vi "WriteLogFile.vi"(4 "Run uninterrupted?":bool, 6 "Automatic warning":string caption="Automatic warning (e.g. large Temperature/RH fluctuations)", 7 "Data File":string, 8 "Error In":errorcluster, 9 "DUT passed?":bool, 10 "Value TechSpec criteria":dbl, 11 "Files saved?":bool) -> (0 "Error Out":errorcluster)   [LabVIEW 2018]
uses:
  globals/QC_RunInformation.vi
panel:
  out "Cause for quitting measurement":string
  in  "OK Button":bool
  in  "Add comment":bool
  out "Type of measurement":string
  out "Logfile entry":string
  # "Write Logfile"
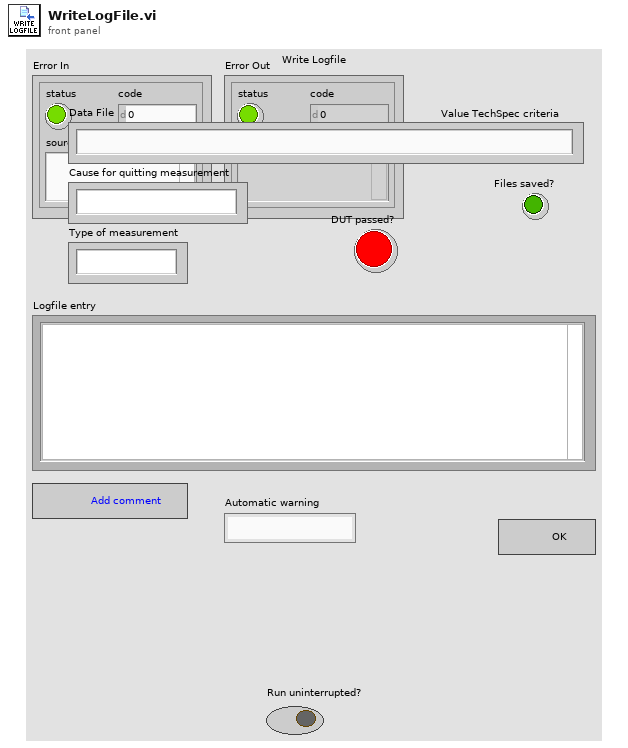
[diagram p1: front panel]
types:
  T1 = enum16{"open", "replace", "create", "open or create", "replace or create", "replace or create with confirmation"}
  T2 = cluster{"Sensor Serial No.:":string, "Wafer:":string, "Batch:":string, "Manufacturer:":string, "Device Category:":string, "Database Serial No.:":string, "Date Initiated:":string, "Time Initiated:":string, "Test":string, "Probeplan used:":string, "End of Run Status":dbl, "End of Run comment:":string, "User:":string, "Vbias SMU":string, "LCR":string, "Test SMU":string, "Test DMM":string, "Comments":string, "Measurement results":cluster{"IV":string, "CV":string, "Cis":string, "Ris":string, "Stability":string, "PTP":string, "Striptest":string}}
  T3 = cluster{"Institute":string, "Manufacturers":string[], "Devices":string[], "Serialnumbers Lookup DB":string, "Data directory":string, "Backup & screenshot directory":string, "List of known users":string[], "Measurement switch not used":bool, "Measurement Switch":string, "DUT Switch":string, "Rseries IV [MOhm]":string, "Rshunt IV [MOhm]":string, "Rseries CV [MOhm]":string, "DC blocking Cap [µF]":string, "Rseries LCR [MOhm]":string, "Rseries stability [MOhm]":string, "Rshunt stability [MOhm]":string, "Rseries striptest bias [MOhm]":string, "Rseries strip pinhole [MOhm]":string}
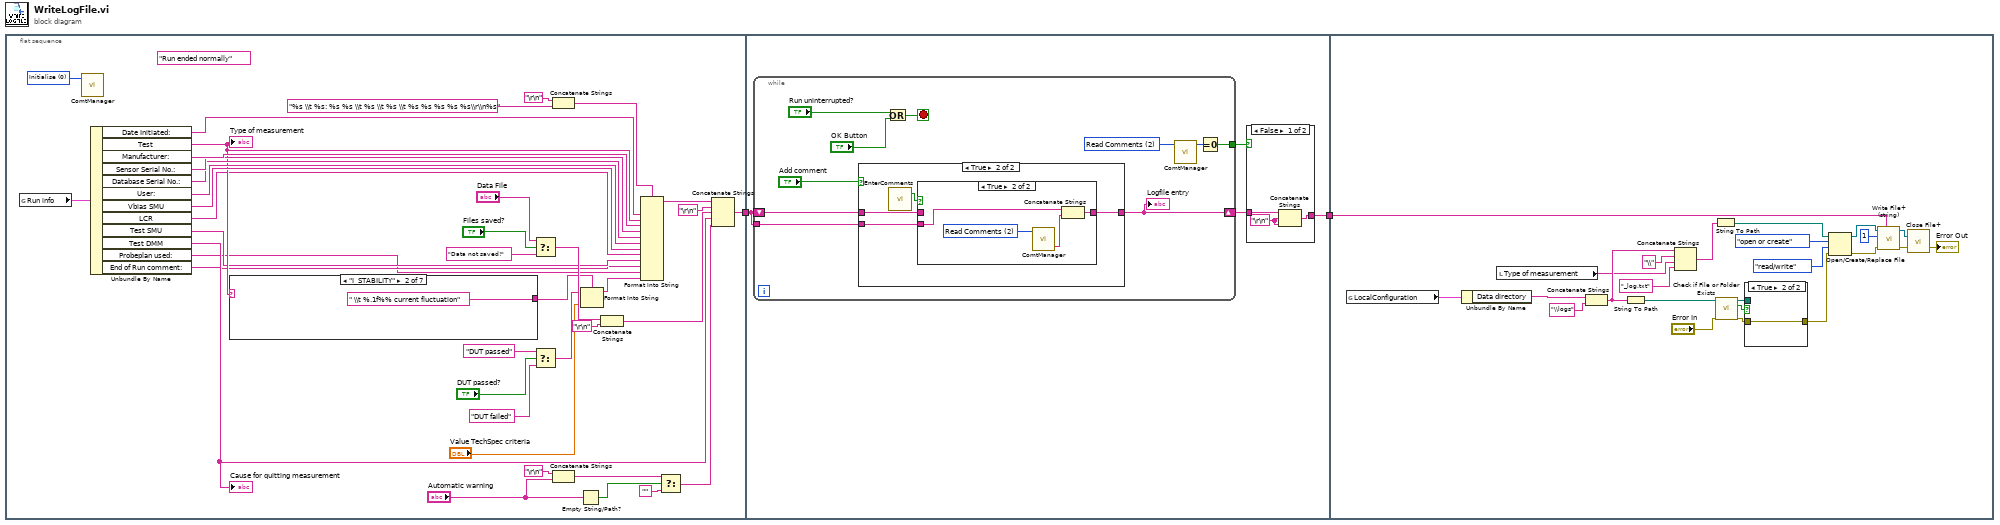
[diagram p0: block diagram]
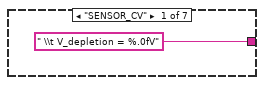
[diagram p2: hidden frame]
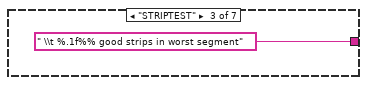
[diagram p3: hidden frame]
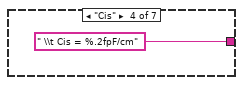
[diagram p4: hidden frame]
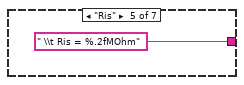
[diagram p5: hidden frame]
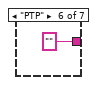
[diagram p6: hidden frame]
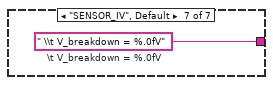
[diagram p7: hidden frame]
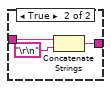
[diagram p8: hidden frame]
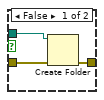
[diagram p11: hidden frame]
diagram:
  n1 = flat-sequence {
    tunnel: [w35] -> w2
    tunnel: w2 -> [w52]
    tunnel: [w50] -> w1
    tunnel: w1 -> [w94]
    frame #0 {
      (unwired) "Run ended normally" ("Cause for quitting measurement")
      w34 = u16 0 items=["Initialise", "Add comment", "Read Comments"] ("Action")
      n2 = global read "QC_RunInformation.vi" "Run info"() -> (w33:T2)
      n3 = call "ComtManager.vi"("Action"=w34) -> ()  [unwired: 2 in, 3 out]
      n4 = Unbundle By Name(w33) -> ("Date Initiated:"=w41:string, "Test"=w16:string, "Manufacturer:"=w31:string, "Sensor Serial No.:"=w30:string, "Database Serial No.:"=w29:string, "User:"=w28:string, "Vbias SMU"=w27:string, "LCR"=w7:string, "Test SMU"=w6:string, "Test DMM"=w5:string, "Probeplan used:"=w4:string, "End of Run comment:"=w18:string)
      "Type of measurement" <- w16
      "Cause for quitting measurement" <- w18
      n5 = case shown="\"I_STABILITY\"" w16 {
        tunnel: [" \\t V_depletion = %.0fV" " \\t %.1f%% current fluctuation" " \\t %.1f%% good strips in worst segment" " \\t Cis = %.2fpF/cm" " \\t Ris = %.2fMOhm" "" w48] -> w15
        frame "SENSOR_CV" {
        }
        frame "I_STABILITY" {
        }
        frame "STRIPTEST" {
        }
        frame "Cis" {
        }
        frame "Ris" {
        }
        frame "PTP" {
        }
        frame "SENSOR_IV", Default {
          w48 = " \\t V_breakdown = %.0fV"  # \t V_breakdown = %.0fV
        }
      }
      n6 = Select(t="Data File", s="Files saved?", f="Data not saved!") -> (s? t:f=w20:string)
      n7 = Select(t="DUT passed", s="DUT passed?", f="DUT failed") -> (s? t:f=w14:string)
      n8 = Concatenate Strings("\r\n", "%s \\t %s: %s %s \\t %s \\t %s \\t %s %s %s %s %s\\r\\n%s") -> (w39:string)
      n9 = Concatenate Strings("\r\n", "Automatic warning") -> (w10:string)
      n10 = Empty String/Path?(string/path="Automatic warning") -> (empty?=w12:bool)
      n11 = Format Into String(format string=w15, initial string=w14, "Value TechSpec criteria") -> (resulting string=w3:string)  [unwired: 1 in, 1 out]
      n12 = Concatenate Strings(w20, "\r\n") -> (w36:string)
      n13 = Format Into String(format string=w39, w41, w16, w31, w30, w29, w28, w27, w7, w6, w5, w4, w3) -> (resulting string=w37:string)  [unwired: 2 in, 1 out]
      n14 = Select(t=w10, s=w12, f="") -> (s? t:f=w8:string)
      n15 = Concatenate Strings(w37, "\r\n", w36, w18, w8) -> (w35:string)
    }
    frame #1 {
      n16 = while {
        shift-right: [w65] -> w51
        shift-left: w52 -> [w67]
        tunnel: w52 -> [w66]
        tunnel: [w62] -> w49
        stop <- w59 stop-if-true
        w64 = u16 2 items=["Initialise", "Add comment", "Read Comments"] ("Action")
        n17 = case shown="True" "Add comment" {
          tunnel: [w69 w72] -> w65
          tunnel: w67 -> [w69 w71]
          tunnel: w66 -> [_ w70]
          frame False {
          }
          frame True {
            n18 = call "EnterComments.vi"() -> ("update?"=w73:bool)  [unwired: 4 in]
            n19 = case shown="True" w73 {
              tunnel: [w74 w77] -> w72
              tunnel: w71 -> [w74 _]
              tunnel: w70 -> [_ w76]
              frame False {
              }
              frame True {
                w78 = u16 2 items=["Initialise", "Add comment", "Read Comments"] ("Action")
                n20 = call "ComtManager.vi"("Action"=w78) -> ("Comment out"=w75:string)  [unwired: 2 in, 2 out]
                n21 = Concatenate Strings(w76, w75) -> (w77:string)
              }
            }
          }
        }
        "Logfile entry" <- w65
        n22 = Or(x="Run uninterrupted?", y="OK Button") -> (x .or. y?=w59:bool)
        n23 = call "ComtManager.vi"("Action"=w64) -> ("No of comments"=w63:i32)  [unwired: 2 in, 2 out]
        n24 = Equal To 0?(x=w63) -> (x = 0?=w62:bool)
      }
      n25 = case shown="False" w49 {
        tunnel: w51 -> [w53 w57]
        tunnel: [w54 w56] -> w50
        frame False {
          w55 = "\r\n"
          n26 = Concatenate Strings(w53, w55, w55) -> (w54:string)
        }
        frame True {
          n27 = Concatenate Strings(w57, "\r\n") -> (w56:string)
        }
      }
    }
    frame #2 {
      n28 = global read "QC_RunInformation.vi" "LocalConfiguration"() -> (w93:T3)
      n29 = Unbundle By Name(w93) -> ("Data directory"=w91:string)
      n30 = local read "Type of measurement"() -> (w79:string)
      n31 = Concatenate Strings(w91, "\\logs") -> (w88:string)
      n32 = String To Path(string=w88) -> (path=w85:path)
      n33 = Concatenate Strings(w88, "\\", w79, "_log.txt") -> (w87:string)
      n34 = String To Path(string=w87) -> (path=w86:path)
      n35 = call <vilib>:"Check if File or Folder Exists.vi"("error in (no error)"="Error In", "path"=w85) -> ("error out"=w81:errorcluster, "file or folder exists?"=w84:bool, "dup path"=w83:path)  [unwired: 7 in]
      n36 = case shown="True" w84 {
        tunnel: w83 -> [w105 _]
        tunnel: w81 -> [w104 w106]
        tunnel: [w103 w106] -> w80
        frame False {
          n37 = Create Folder(path (use dialog)=w105, error in=w104) -> (error out=w103:errorcluster)  [unwired: 1 in, 2 out]
        }
        frame True {
        }
      }
      n38 = Open/Create/Replace File(file path (use dialog)=w86, error in=w80, operation (0:open)=T1."open or create", access (0:read/write)=enum16{"read/write", "read-only", "write-only"}."read/write") -> (refnum out=w99:refnum<file>, error out=w100:errorcluster)  [unwired: 2 in, 1 out]
      n39 = call <vilib>:"Write File+ (string).vi"("string"=w94, "error in (no error)"=w100, "pos mode (rel. to end:1)"=1, "refnum"=w99) -> ("error out"=w96:errorcluster, "dup refnum"=w95:refnum<file>)  [unwired: 3 in, 1 out]
      n40 = call <vilib>:"Close File+.vi"("error in (no error)"=w96, "refnum"=w95) -> ("error out"=→"Error Out":errorcluster)  [unwired: 3 in, 2 out]
    }
  }
